vi "Define_Indicies_of_Affected_Subtracks-1.vi"(0 "[IN] Subtracks":T2(array[cluster]), 1 "[IN] # of Prob\nlem Point Inside":i32, 3 "[IN] # of Longest track\nInside the Group of Tracks":i32, 5 "[IN] Index of connected \npoints inside the track":i32[](array[numeric]), 9 "[IN] Index of # tracks \nwith problem points":i32[](array[numeric]), 11 "error IN":errorcluster, 12 "[IN] Status of 1st Problem Point":i16, 14 "[IN] Values for Cost F() Calc":T1) -> (4 "[OUT] Indicies of \nPoints Inside Trks":i32[](array[numeric]), 6 "[OUT] Indicies of \nall Affected Tracks\n(initial point =0)":i32[](array[numeric]), 8 "[OUT] Index of Optimal \nSubtrack Splitting Case":i32, 10 "[OUT] Optimal solution \nfor Merging Case":i32[](array[numeric]), 15 "error OUT":errorcluster)   [LabVIEW 2013]
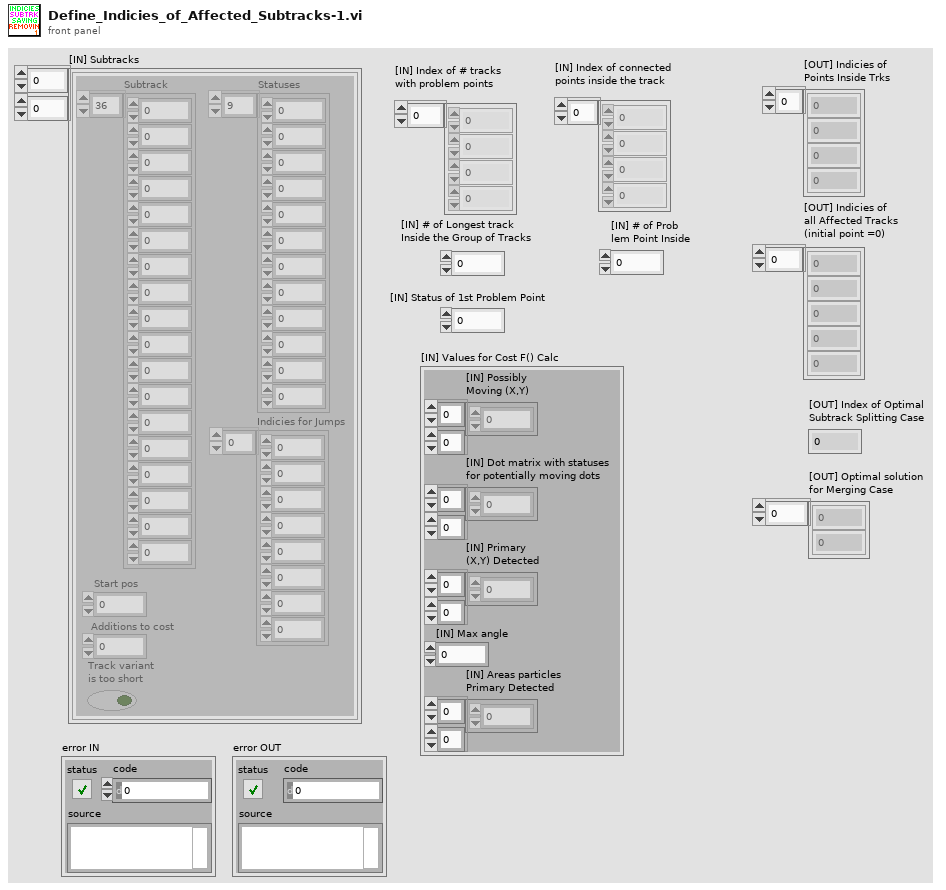
[diagram p1: front panel]
types:
  T1 = cluster{"[IN] Possibly\nMoving (X,Y)":dbl[][], "[IN] Dot matrix with statuses \nfor potentially moving dots":i16[][], "[IN] Primary \n(X,Y) Detected ":dbl[][], "[IN] Max angle":dbl, "[IN] Areas particles\nPrimary Detected ":dbl[][]}
  T2 = cluster{"Subtrack":dbl[], "Statuses":i16[], "Start pos":i32, "Additions to cost":i8, "Track variant \nis too short":bool, "Indicies for Jumps":i32[]}[][]
  T3 = cluster{"Subtrack":dbl[], "Statuses":i16[], "Start pos":i32, "Additions to cost":i8, "Track variant \nis too short":bool, "Indicies for Jumps":i32[]}[]
  T4 = cluster{"Subtrack":dbl[], "Statuses":i16[], "Start pos":i32, "Additions to cost":i8, "Track variant \nis too short":bool, "Indicies for Jumps":i32[]}
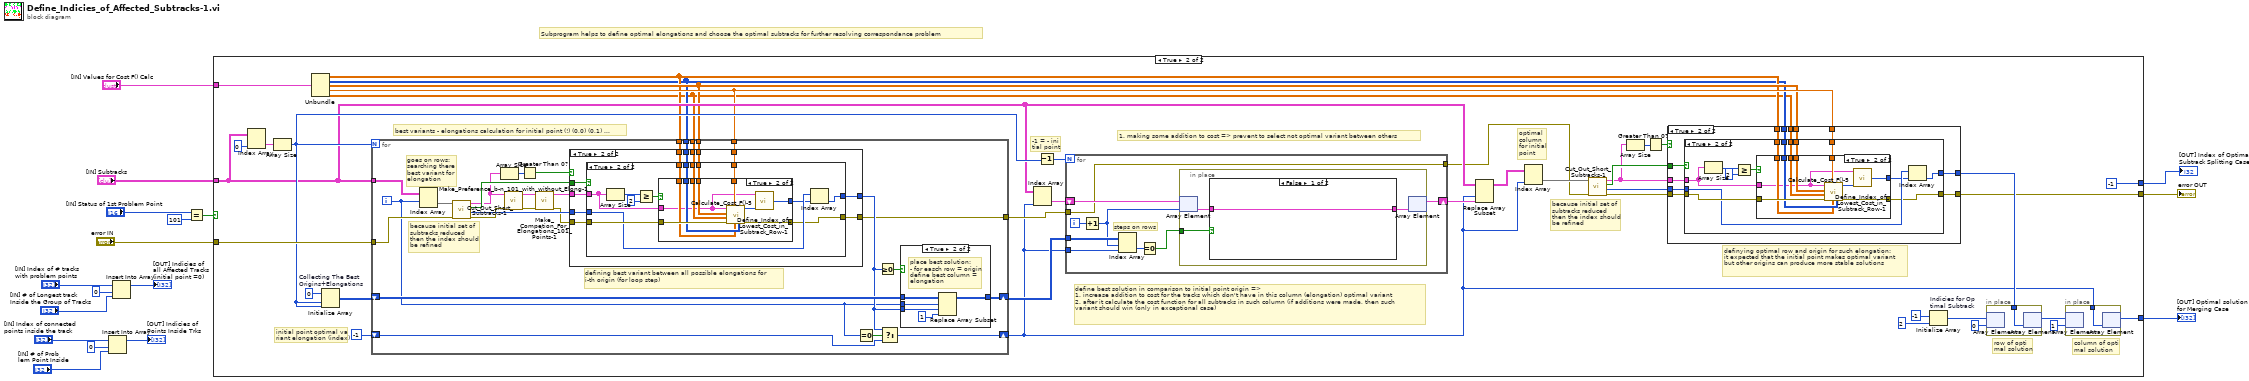
[diagram p0: block diagram]
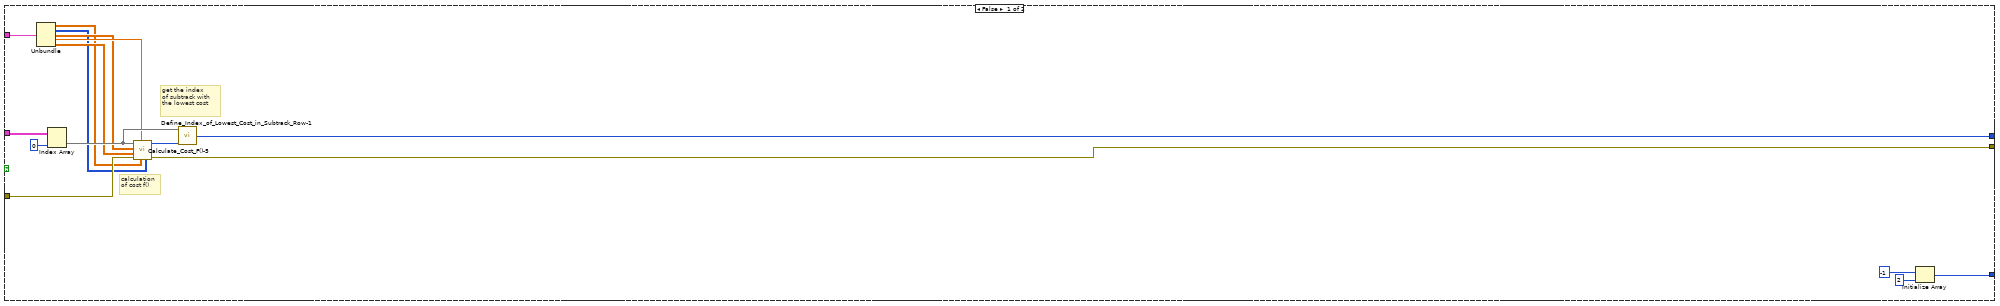
[diagram p2: hidden frame]
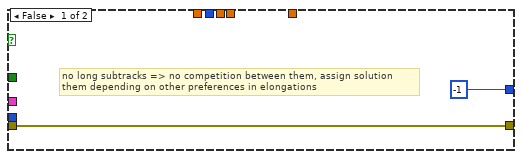
[diagram p3: hidden frame]
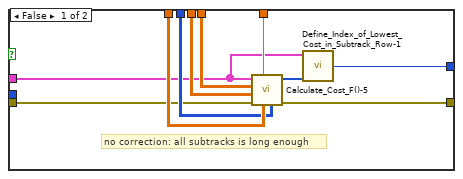
[diagram p4: hidden frame]
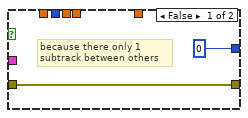
[diagram p5: hidden frame]
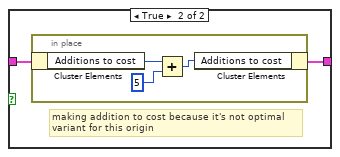
[diagram p6: hidden frame]
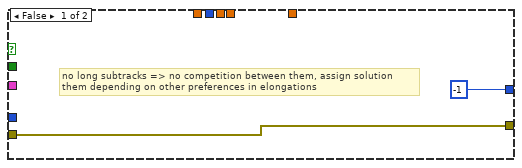
[diagram p8: hidden frame]
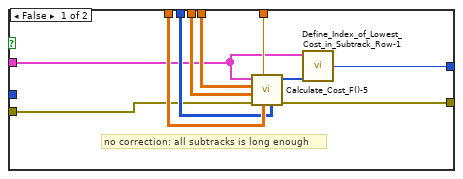
[diagram p9: hidden frame]
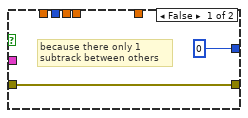
[diagram p10: hidden frame]
diagram:
  # "Subprogram helps to define optimal elongations and choose the optimal subtracks for further resolving correspondance problem"
  n1 = Insert Into Array(array="[IN] Index of connected \npoints inside the track", index=0, new element="[IN] # of Prob\nlem Point Inside") -> (→"[OUT] Indicies of \nPoints Inside Trks":i32[])
  n2 = Insert Into Array(array="[IN] Index of # tracks \nwith problem points", index=0, new element="[IN] # of Longest track\nInside the Group of Tracks") -> (→"[OUT] Indicies of \nall Affected Tracks\n(initial point =0)":i32[])
  n3 = Equal?(x="[IN] Status of 1st Problem Point", y=i16 101) -> (x = y?=w15:bool)
  n4 = case shown="True" w15 {
    tunnel: "[IN] Subtracks" -> [w33 w61]
    tunnel: "error IN" -> [w31 w68]
    tunnel: "[IN] Values for Cost F() Calc" -> [w28 w67]
    tunnel: [w18 w36] -> w8
    tunnel: [w21 w35] -> w7
    tunnel: [w22 -1 ("[OUT] Index of Optimal Subtrack")] -> w6
    frame False {
      # "get the index \nof subtrack with \nthe lowest cost"
      # "calculation \nof cost f()"
      n5 = Unbundle(w28) -> ("[IN] Possibly\nMoving (X,Y)"=w24:dbl[][], "[IN] Dot matrix with statuses \nfor potentially moving dots"=w23:i16[][], "[IN] Primary \n(X,Y) Detected"=w25:dbl[][], "[IN] Max angle"=w26:dbl, "[IN] Areas particles\nPrimary Detected"=w27:dbl[][])
      n6 = Index Array(array=w33, index (col)=0 ("disabled index (col)")) -> (element=w29:T3)  [unwired: 1 in]
      n7 = call "Calculate_Cost_F()-5.vi"("[IN] Dot matrix with statuses \nfor potentially moving dots"=w23, "[IN] Potentially\nMoving (X,Y)"=w24, "[IN] Max angle"=w26, "error IN"=w31, "[IN] Areas particles\nPrimary Detected"=w27, "[IN] Primary \n(X,Y) Detected"=w25, "[IN] Subtracks in Row"=w29) -> ("error OUT"=w21:errorcluster, "[OUT] Cost function"=w30:i8[])  [unwired: 3 in]
      n8 = call "Define_Index_of_Lowest_Cost_in_Subtrack_Row-1.vi"("[IN] Cost functions"=w30, "[IN] Subtracks in Row"=w29) -> ("[OUT] Index of Optimal Subtrack"=w22:i32)  [unwired: 4 in]
      n9 = Initialize Array(-1 ("element"), 2 ("dimension size")) -> (w18:i32[])
    }
    frame True {
      # "column of opti\nmal solution"
      # "row of opti\nmal solution"
      # "optimal \ncolumn \nfor initial\npoint"
      # "because initial set of \nsubtracks reduced \nthen the index should \nbe refined"
      # "definying optimal row and origin for such elongation: \nit expected that the initial point makes optimal variant\nbut other origins can produce more stable solutions"
      # "1. making some addition to cost => prevent to select not optimal variant between others"
      # "-1 = - ini\ntial point"
      # "initial point optimal va\nriant elongation (index)"
      # "define best solution in comparison to initial point origin =>\n1. increase addition to cost for the tracks which don't have in this column (elongation) optimal variant\n2. after it calculate the cost function for all subtracks in such column (if additions were made, then such \nvariant should win (only in exceptional case)"
      # "best variants - elongations calculation for initial point (!) (0,0) (0,1) ..."
      n10 = Index Array(array=w61, index (col)=0 ("disabled index (col)")) -> (element=w71:T3)  [unwired: 1 in]
      n11 = Array Size(array=w71) -> (size(s)=w65:i32)
      n12 = Unbundle(w67) -> ("[IN] Possibly\nMoving (X,Y)"=w47:dbl[][], "[IN] Dot matrix with statuses \nfor potentially moving dots"=w46:i16[][], "[IN] Primary \n(X,Y) Detected"=w48:dbl[][], "[IN] Max angle"=w49:dbl, "[IN] Areas particles\nPrimary Detected"=w45:dbl[][])
      n13 = Initialize Array "Collecting The Best \nOrigins+Elongations"(0 ("element"), w65, w65) -> (w69:i32[][])
      n14 = for {
        N: w65 -> [_]
        shift-right: [w154] -> w62
        shift-left: w69 -> [w155]
        tunnel: w61 -> [w163]
        tunnel: w68 -> [w162]
        tunnel: w49 -> [w161]
        tunnel: w48 -> [w160]
        tunnel: w45 -> [w159]
        tunnel: w47 -> [w158]
        tunnel: w46 -> [w157]
        shift-right: [w152] -> w37
        shift-left: -1 -> [w149]
        tunnel: [w148] -> w51
        i -> [w151]
        # "because initial set of \nsubtracks reduced \nthen the index should \nbe refined"
        # "goes on rows:\nsearching there \nbest variant for \nelongation"
        # "defining best variant between all possible elongations for \ni-th origin (for loop step)"
        n15 = Index Array(array=w163, index (row)=w151) -> (element=w168:T3)  [unwired: 1 in]
        n16 = call "Cut_Out_Short_Subtracks-1.vi"("error IN"=w162, "[IN] Subtracks in Row"=w168) -> ("error OUT"=w146:errorcluster, "[OUT] Indicies of subttracks\nin initial row with them"=w166:i32[], "[OUT] Some tracks are empty"=w167:bool, "[OUT Subtracks in Row"=w147:T3)  [unwired: 2 in]
        n17 = Array Size(array=w147) -> (size(s)=w165:i32)
        n18 = call "Make_Preference_b-n_101_with_without_Elong-1.vi"("error IN"=w146, "[IN] Subtracks in Row"=w147) -> ("error OUT"=w143:errorcluster, "[OUT Subtracks in Row"=w145:T3)  [unwired: 4 in]
        n19 = Greater Than 0?(x=w165) -> (x > 0?=w164:bool)
        n20 = call "Make_Competion_For_Elongations_101_Points-1.vi"("error IN"=w143, "[IN] Subtracks in Row"=w145) -> ("error OUT"=w142:errorcluster, "[OUT Subtracks in Row"=w144:T3)  [unwired: 4 in]
        n21 = case shown="True" w164 {
          tunnel: w161 -> [_ w187]
          tunnel: w160 -> [_ w186]
          tunnel: w159 -> [_ w185]
          tunnel: w158 -> [_ w184]
          tunnel: w157 -> [_ w183]
          tunnel: [w176 w182] -> w148
          tunnel: w144 -> [_ w181]
          tunnel: w142 -> [w176 w180]
          tunnel: w167 -> [_ w179]
          tunnel: [-1 ("element") w178] -> w153
          tunnel: w166 -> [_ w177]
          frame False {
            # "no long subtracks => no competition between them, assign solution\nthem depending on other preferences in elongations"
          }
          frame True {
            n22 = case shown="True" w179 {
              tunnel: w187 -> [w197 w204]
              tunnel: w186 -> [w196 w205]
              tunnel: w185 -> [w195 w206]
              tunnel: w184 -> [w194 w208]
              tunnel: w183 -> [w193 w207]
              tunnel: [w191 w198] -> w182
              tunnel: w181 -> [w190 w203]
              tunnel: w180 -> [w189 w202]
              tunnel: [w188 w199] -> w178
              tunnel: w177 -> [_ w201]
              frame False {
                # "no correction: all subtracks is long enough"
                n23 = call "Calculate_Cost_F()-5.vi"("[IN] Dot matrix with statuses \nfor potentially moving dots"=w193, "[IN] Potentially\nMoving (X,Y)"=w194, "[IN] Max angle"=w197, "error IN"=w189, "[IN] Areas particles\nPrimary Detected"=w195, "[IN] Primary \n(X,Y) Detected"=w196, "[IN] Subtracks in Row"=w190) -> ("error OUT"=w191:errorcluster, "[OUT] Cost function"=w192:i8[])  [unwired: 3 in]
                n24 = call "Define_Index_of_Lowest_Cost_in_Subtrack_Row-1.vi"("[IN] Cost functions"=w192, "[IN] Subtracks in Row"=w190) -> ("[OUT] Index of Optimal Subtrack"=w188:i32)  [unwired: 4 in]
              }
              frame True {
                n25 = Array Size(array=w203) -> (size(s)=w211:i32)
                n26 = Greater Or Equal?(x=w211, y=2) -> (x >= y?=w209:bool)
                n27 = case shown="True" w209 {
                  tunnel: w208 -> [_ w217]
                  tunnel: w207 -> [_ w218]
                  tunnel: w206 -> [_ w219]
                  tunnel: w205 -> [_ w220]
                  tunnel: w204 -> [_ w221]
                  tunnel: w203 -> [_ w216]
                  tunnel: w202 -> [w212 w222]
                  tunnel: [w212 w215] -> w198
                  tunnel: [0 w214] -> w200
                  frame False {
                    # "because there only 1 \nsubtrack between others"
                  }
                  frame True {
                    n28 = call "Calculate_Cost_F()-5.vi"("[IN] Dot matrix with statuses \nfor potentially moving dots"=w218, "[IN] Potentially\nMoving (X,Y)"=w217, "[IN] Max angle"=w221, "error IN"=w222, "[IN] Areas particles\nPrimary Detected"=w219, "[IN] Primary \n(X,Y) Detected"=w220, "[IN] Subtracks in Row"=w216) -> ("error OUT"=w215:errorcluster, "[OUT] Cost function"=w223:i8[])  [unwired: 3 in]
                    n29 = call "Define_Index_of_Lowest_Cost_in_Subtrack_Row-1.vi"("[IN] Cost functions"=w223, "[IN] Subtracks in Row"=w216) -> ("[OUT] Index of Optimal Subtrack"=w214:i32)  [unwired: 4 in]
                  }
                }
                n30 = Index Array(array=w201, index=w200) -> (element=w199:i32)
              }
            }
          }
        }
        n31 = Equal To 0?(x=w151) -> (x = 0?=w150:bool)
        n32 = Greater Or Equal To 0?(x=w153) -> (x >= 0?=w156:bool)
        n33 = Select(t=w153, s=w150, f=w149) -> (s? t:f=w152:i32)
        n34 = case shown="True" w156 {
          tunnel: w155 -> [w169 w174]
          tunnel: w151 -> [_ w173]
          tunnel: w153 -> [_ w172]
          tunnel: [w169 w170] -> w154
          frame False {
          }
          frame True {
            # "place best solution:\n- for easch row = origin\ndefine best column =\nelongation"
            n35 = Replace Array Subset(array=w174, new element=1 ("new element/subarray"), index (row)=w173, index (col)=w172) -> (w170:i32[][])
          }
        }
      }
      n36 = Index Array(array=w61, index (col)=w37) -> (element=w63:T3)  [unwired: 1 in]
      n37 = Decrement(x=w65) -> (x-1=w64:i32)
      n38 = for {
        N: w64 -> [_]
        shift-right: [w125] -> w60
        shift-left: w63 -> [w129]
        tunnel: w62 -> [w131]
        tunnel: w37 -> [w130]
        tunnel: w51 -> [w124]
        tunnel: [w124] -> w50
        i -> [w132]
        # "steps on rows"
        n39 = Increment(x=w132) -> (x+1=w128:i32)
        n40 = Index Array(array=w131, index (row)=w128, index (col)=w130) -> (element=w127:i32)
        n41 = Equal To 0?(x=w127) -> (x = 0?=w126:bool)
        n42 = in-place {
          in-place-border: w126 -> [w135]
          n43 = in-place-array #1(w129, w128) -> (w134:T4)
          n44 = case shown="False" w135 {
            tunnel: w134 -> [w136 w138]
            tunnel: [w136 w137] -> w133
            frame False {
            }
            frame True {
              # "making addition to cost because it's not optimal\nvariant for this origin"
              n45 = in-place {
                n46 = in-place-cluster #2(w138) -> ("Additions to cost"=w141:i8)
                n47 = Add(x=w141, y=i8 5) -> (x+y=w139:i8)
                n48 = in-place-cluster #2("Additions to cost"=w139) -> (w137:T4)
              }
            }
          }
          n49 = in-place-array #1(w133) -> (w125:T3)  [unwired: 1 out]
        }
      }
      n50 = Replace Array Subset(array=w61, new element=w60, index (col)=w37) -> (w53:T2)  [unwired: 1 in]
      n51 = Index Array(array=w53, index (col)=w37) -> (element=w52:T3)  [unwired: 1 in]
      n52 = call "Cut_Out_Short_Subtracks-1.vi"("error IN"=w50, "[IN] Subtracks in Row"=w52) -> ("error OUT"=w59:errorcluster, "[OUT] Indicies of subttracks\nin initial row with them"=w57:i32[], "[OUT] Some tracks are empty"=w58:bool, "[OUT Subtracks in Row"=w56:T3)  [unwired: 2 in]
      n53 = Array Size(array=w56) -> (size(s)=w55:i32)
      n54 = Greater Than 0?(x=w55) -> (x > 0?=w54:bool)
      n55 = case shown="True" w54 {
        tunnel: w49 -> [_ w87]
        tunnel: w48 -> [_ w86]
        tunnel: w45 -> [_ w85]
        tunnel: w47 -> [_ w84]
        tunnel: w46 -> [_ w83]
        tunnel: [w76 w82] -> w35
        tunnel: w56 -> [_ w81]
        tunnel: w59 -> [w76 w80]
        tunnel: w58 -> [_ w79]
        tunnel: [-1 ("element") w78] -> w40
        tunnel: w57 -> [_ w77]
        frame False {
          # "no long subtracks => no competition between them, assign solution\nthem depending on other preferences in elongations"
        }
        frame True {
          n56 = case shown="True" w79 {
            tunnel: w87 -> [w97 w104]
            tunnel: w86 -> [w96 w105]
            tunnel: w85 -> [w95 w106]
            tunnel: w84 -> [w94 w108]
            tunnel: w83 -> [w93 w107]
            tunnel: [w91 w98] -> w82
            tunnel: w81 -> [w90 w103]
            tunnel: w80 -> [w89 w102]
            tunnel: [w88 w99] -> w78
            tunnel: w77 -> [_ w101]
            frame False {
              # "no correction: all subtracks is long enough"
              n57 = call "Calculate_Cost_F()-5.vi"("[IN] Dot matrix with statuses \nfor potentially moving dots"=w93, "[IN] Potentially\nMoving (X,Y)"=w94, "[IN] Max angle"=w97, "error IN"=w89, "[IN] Areas particles\nPrimary Detected"=w95, "[IN] Primary \n(X,Y) Detected"=w96, "[IN] Subtracks in Row"=w90) -> ("error OUT"=w91:errorcluster, "[OUT] Cost function"=w92:i8[])  [unwired: 3 in]
              n58 = call "Define_Index_of_Lowest_Cost_in_Subtrack_Row-1.vi"("[IN] Cost functions"=w92, "[IN] Subtracks in Row"=w90) -> ("[OUT] Index of Optimal Subtrack"=w88:i32)  [unwired: 4 in]
            }
            frame True {
              n59 = Array Size(array=w103) -> (size(s)=w111:i32)
              n60 = Greater Or Equal?(x=w111, y=2) -> (x >= y?=w109:bool)
              n61 = case shown="True" w109 {
                tunnel: w108 -> [_ w117]
                tunnel: w107 -> [_ w118]
                tunnel: w106 -> [_ w119]
                tunnel: w105 -> [_ w120]
                tunnel: w104 -> [_ w121]
                tunnel: w103 -> [_ w116]
                tunnel: w102 -> [w112 w122]
                tunnel: [w112 w115] -> w98
                tunnel: [0 w114] -> w100
                frame False {
                  # "because there only 1 \nsubtrack between others"
                }
                frame True {
                  n62 = call "Calculate_Cost_F()-5.vi"("[IN] Dot matrix with statuses \nfor potentially moving dots"=w118, "[IN] Potentially\nMoving (X,Y)"=w117, "[IN] Max angle"=w121, "error IN"=w122, "[IN] Areas particles\nPrimary Detected"=w119, "[IN] Primary \n(X,Y) Detected"=w120, "[IN] Subtracks in Row"=w116) -> ("error OUT"=w115:errorcluster, "[OUT] Cost function"=w123:i8[])  [unwired: 3 in]
                  n63 = call "Define_Index_of_Lowest_Cost_in_Subtrack_Row-1.vi"("[IN] Cost functions"=w123, "[IN] Subtracks in Row"=w116) -> ("[OUT] Index of Optimal Subtrack"=w114:i32)  [unwired: 4 in]
                }
              }
              n64 = Index Array(array=w101, index=w100) -> (element=w99:i32)
            }
          }
        }
      }
      n65 = Initialize Array "Indicies for Op\ntimal Subtrack"(-1 ("element"), 2 ("dimension size")) -> (w42:i32[])
      n66 = in-place {
        in-place-border: w40 -> [w74]
        n67 = in-place-array #3(w42, 0) -> ()  [unwired: 1 out]
        n68 = in-place-array #3(w74) -> (w38:i32[])  [unwired: 1 out]
      }
      n69 = in-place {
        in-place-border: w37 -> [w73]
        n70 = in-place-array #4(w38, 1) -> ()  [unwired: 1 out]
        n71 = in-place-array #4(w73) -> (w36:i32[])  [unwired: 1 out]
      }
    }
  }
  "error OUT" <- w7
  "[OUT] Optimal solution \nfor Merging Case" <- w8
  "[OUT] Index of Optimal \nSubtrack Splitting Case" <- w6
